vi "Auton Script Builder.vi"   [LabVIEW 2015]
uses:
  Robot Global Data.vi
  <vilib>/Utility/file.llb/Read Delimited Spreadsheet (DBL).vi
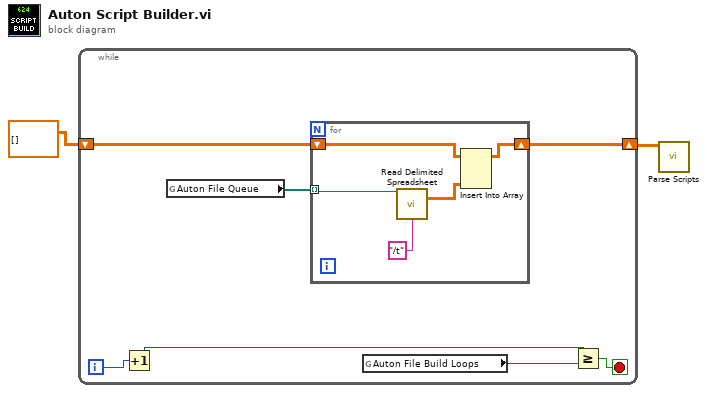
[diagram p0: block diagram]
diagram:
  n1 = while {
    shift-right: [w3] -> w1
    shift-left: dbl[][] [] -> [w4]
    i -> [w8]
    stop <- w6 stop-if-true
    n2 = Increment(x=w8) -> (x+1=w7:i32)
    n3 = global read "Robot Global Data.vi" "Auton File Queue"() -> (w9:path[])
    n4 = for {
      tunnel: w9 -> [w14] mode=indexing
      shift-right: [w11] -> w3
      shift-left: w4 -> [w13]
      n5 = call-poly <vilib>:"Read Delimited Spreadsheet.vi"("file path (dialog if empty)"=w14, "delimiter (\\t)"="/t" ("delimiter (\\t)")) -> ("all rows"=w12:dbl[][])  [unwired: 8 in, 5 out]
      n6 = Insert Into Array(array=w13, new element=w12) -> (w11:dbl[][])  [unwired: 2 in]
    }
    n7 = global read "Robot Global Data.vi" "Auton File Build Loops"() -> (w5:i32)
    n8 = Greater Or Equal?(x=w7, y=w5) -> (x >= y?=w6:bool)
  }
  n9 = call "Parse Scripts.vi"("Array"=w1) -> ()  [unwired: 11 in]
